vi "Module Init.vi"(8 "error in (no error)":errorcluster, 11 "Config Updater Module in":refnum<class "Git Updater Module.lvclass">) -> (0 "error out":errorcluster, 3 "Config Updater Module out":refnum<class "Git Updater Module.lvclass">)   [LabVIEW 2020, in "Volatus.lvlib" / "Git Updater Module.lvclass"]
uses:
  Git Updater Module.lvclass
  Git Updater Module.lvclass/Git Updater Module.ctl
  Module/Module.lvclass
  C:/dev/lv20CE/relink/lv-volatus/Volatus/Module/Module.lvclass
  C:/dev/lv20CE/relink/lv-volatus/Volatus/Git Updater Module/Git Updater Module.lvclass
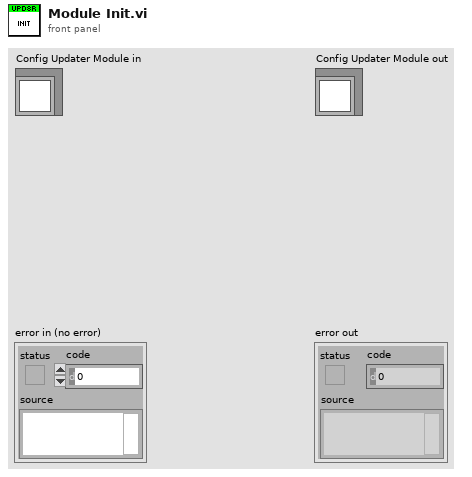
[diagram p1: front panel]
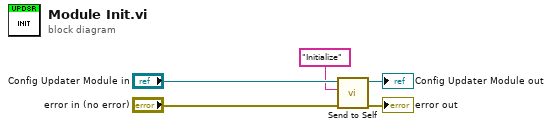
[diagram p0: block diagram]
diagram:
  n1 = call "Send to Self.vi"("error in (no error)"="error in (no error)", "Message ID"="Initialize", "Module in"="Config Updater Module in") -> ("error out"=→"error out":errorcluster, "Module out"=→"Config Updater Module out":refnum<class "Git Updater Module.lvclass">)  [unwired: 7 in]
